vi "Do.vi"(8 "error in":errorcluster, 10 "Actor in":refnum<class "Actor.lvclass">, 11 "Enable Compressor MSG":refnum<class "Enable Fan MSG.lvclass">) -> (0 "error out":errorcluster, 2 "Actor out":refnum<class "Actor.lvclass">)   [LabVIEW 2017, in "Controller.lvlib" / "Enable Fan MSG.lvclass"]
doc: "(<B>Filename</B>: Actor Framework.lvlib:Message.lvclass:Do.vi)\n\nDefines what a message does when it is received by an actor. Generally, a message instructs an actor to invoke one of its methods. By default, this method does nothing. A child class must override it to define behavior. Create a child class by using the Actor Framework Message Maker dialog box."
uses:
  Enable Fan MSG.lvclass
  U:/sw_repo/For Builds/Nicholas/Controller/Messages/Generic Boolean MSG/Generic Boolean Message.lvclass
  <vilib>/ActorFramework/Actor/Actor.lvclass
  Generic Boolean MSG/Generic Boolean Message.lvclass/Generic Boolean Message.ctl
  Generic Boolean MSG/Read Bool.vi
  gController.lvclass
  <vilib>/rvi/interface/nirviReadWriteControl/nirviReadWriteControl.xnode
  FPGA Ref.ctl
  FPGA Bitfiles/server.lvbitx
  <vilib>/rvi/errors/niLvFpgaMergeErrorWithErrorCode.vi
  <vilib>/rvi/errors/niLvFpgaAdjustHostInterfaceError.vi
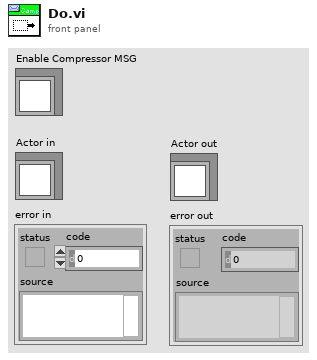
[diagram p1: front panel]
types:
  T1 = typedef "FPGA Ref.ctl" = refnum<k20>
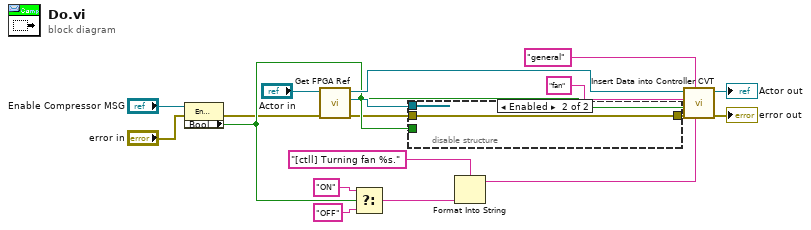
[diagram p0: block diagram]
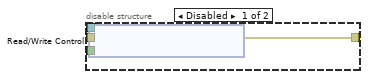
[diagram p2: hidden frame]
diagram:
  n1 = property class="Enable Compressor MSG"(reference="Enable Compressor MSG", error in="error in") -> (error out=w4:errorcluster, "Bool"=w5:bool)  [unwired: 1 out]
  n2 = call "Get FPGA Ref.vi"("error in (no error)"=w4, "Actor In"="Actor in") -> ("error out"=w3:errorcluster, "FPGA Ref"=w6:T1, "Actor Out"=w7:refnum<class "Actor.lvclass">)  [unwired: 7 in]
  n3 = Select(t="ON", s=w5, f="OFF") -> (s? t:f=w11:string)
  n4 = disable-structure shown="Enabled" {
    disable-tunnel: w6 -> [w22 _]
    disable-tunnel: w5 -> [w21 _]
    disable-tunnel: w3 -> [w20 w23]
    disable-tunnel: [w19 w23] -> w2
    frame Disabled {
      n5 = xnode "Read/Write Control"("FPGA VI Reference In"=w22, "error in"=w20, "Fan Enable"=w21) -> ("error out"=w19:errorcluster)  [unwired: 1 out]
    }
    frame Enabled {
    }
  }
  n6 = Format Into String(format string="[ctll] Turning fan %s.", w11) -> (resulting string=w9:string)  [unwired: 2 in, 1 out]
  n7 = call "Insert Data into Controller CVT.vi"("Update MSG"=w9, "Group"="general", "error in"=w2, "Data"=w5, "tag"="fan", "Actor in"=w7) -> ("error out"=→"error out":errorcluster, "Actor Out"=→"Actor out":refnum<class "Actor.lvclass">)  [unwired: 4 in]
